vi "Comm_close 1d cdb waveform.vi"(8 "error in (no error)":errorcluster, 11 "WPL Comm (1D CDB) in":refnum<class "WPL Comm (1D CDB).lvclass">) -> (0 "error out":errorcluster)   [LabVIEW 2020, in "Internal Comm Classes.lvlib" / "WPL Comm (1D CDB).lvclass"]
uses:
  WPL Comm (1D CDB).lvclass
  D:/p4/penguin/lvaddon/Veristand/master/src/LabVIEW/vilib/NI VeriStand/Custom Device Waveform API/Internal Comm Classes/WPL Comm/WPL Comm.lvclass
  WPL Comm.lvclass/WPL Comm.ctl
  WPL Comm (1D CDB).lvclass/WPL Comm (1D CDB).ctl
  WPL Command.ctl
  Set ErrorQ on Variant.vi
  Send WPL Command.vi
  WPL Comm.lvclass
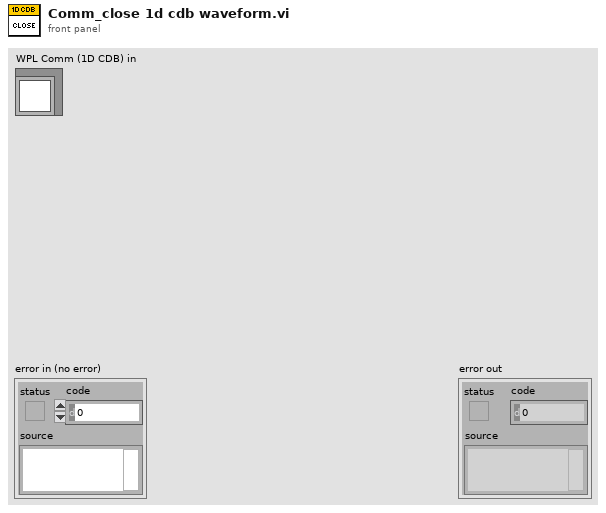
[diagram p1: front panel]
types:
  T1 = typedef "NI_VS Custom Device Waveform API.lvlib/Access mode.ctl" = enum16{"Read", "Write"}
  T2 = typedef "Internal Comm Classes.lvlib/WPL Comm.lvclass/WPL Command.ctl" = enum16{"Register 1D DBL Reader", "Unregister 1D DBL Reader", "Register 1D DBL Writer", "Register 2D DBL Writer", "Unregister 1D DBL Writer", "Unregister 2D DBL Writer", "DBL WFM Start", "WFM 1D DBL Data", "WFM 2D DBL Data", "Shut down", "Handle Error", "Register 1D CDB Reader", "Unregister 1D CDB Reader", "Register 1D CDB Writer", "Unregister 1D CDB Writer", "Register 2D CDB Writer", "Unregister 2D CDB Writer", "WFM 1D CDB Data", "WFM 2D CDB Data", "CDB WFM Start", "Error Shutdown", "Register Streams", "Unregister Streams", "Delete All Streams", "Get WFM DTs", "DBL WFM Multi Start", "CDB WFM Multi Start"}
  T3 = typedef "Internal Comm Classes.lvlib/WPL Comm (1D CDB).lvclass/Waveform 1d cdb read queue.ctl" = refnum<queue>
  T4 = typedef "Internal Comm Classes.lvlib/WPL Comm (1D CDB).lvclass/Waveform 1d cdb queue.ctl" = refnum<queue>
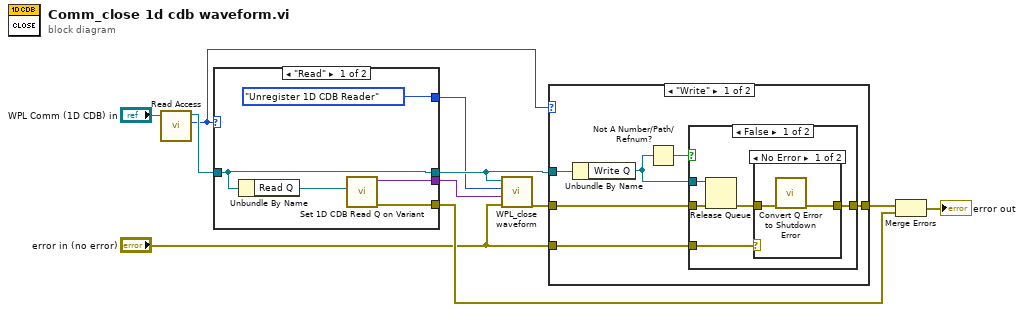
[diagram p0: block diagram]
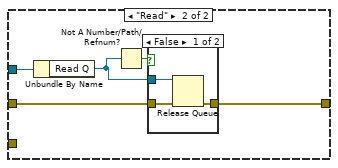
[diagram p4: hidden frame]
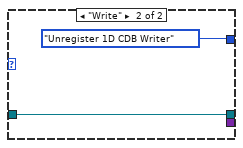
[diagram p6: hidden frame]
diagram:
  n1 = call "Read Access.vi"("WPL Comm in"="WPL Comm (1D CDB) in") -> ("Access"=w6:T1, "WPL Comm out"=w9:refnum<class "WPL Comm (1D CDB).lvclass">)  [unwired: 9 in]
  n2 = case shown="\"Read\"" w6 {
    tunnel: [WPL_Command."Unregister 1D CDB Reader" ("Command") WPL_Command."Unregister 1D CDB Writer" ("Command")] -> w3
    tunnel: w9 -> [w14 w17]
    tunnel: [w14 w17] -> w7
    tunnel: [w15 _] -> w8
    tunnel: [w12 _] -> w2
    frame "Read" {
      n3 = Unbundle By Name(w14) -> ("Read Q"=w13:T3)
      n4 = call "Set 1D CDB Read Q on Variant.vi"("1D CDB Read Q"=w13) -> ("error out"=w15:errorcluster, "Variant out"=w12:variant)  [unwired: 8 in, 1 out]
    }
    frame "Write" {
    }
  }
  n5 = call "WPL_close waveform.vi"("error in (no error)"="error in (no error)", "Variant"=w2, "Command"=w3, "WPL Comm in"=w7) -> ("error out"=w11:errorcluster)  [unwired: 7 in]
  n6 = case shown="\"Write\"" w6 {
    tunnel: w11 -> [w23 w38]
    tunnel: [w20 w37] -> w10
    tunnel: w7 -> [w24 w36]
    tunnel: "error in (no error)" -> [w19 _]
    frame "Write" {
      n7 = Unbundle By Name(w24) -> ("Write Q"=w22:T4)
      n8 = Not A Number/Path/Refnum?(number/path/refnum=w22) -> (NaN/Path/Refnum?=w21:bool)
      n9 = case shown="False" w21 {
        tunnel: w23 -> [w29 w33]
        tunnel: [w26 w33] -> w20
        tunnel: w22 -> [w28 _]
        tunnel: w19 -> [w25 _]
        frame False {
          n10 = Release Queue(queue=w28, error in (no error)=w29) -> (error out=w27:errorcluster)  [unwired: 1 in, 2 out]
          n11 = case shown="No Error" w25 {
            tunnel: w27 -> [w31 w32]
            tunnel: [w30 w32] -> w26
            frame No Error {
              n12 = call "Convert Q Error to Shutdown Error.vi"("error in (no error)"=w31) -> ("error out"=w30:errorcluster)  [unwired: 10 in]
            }
            frame Error {
            }
          }
        }
        frame True {
        }
      }
    }
    frame "Read" {
      n13 = Unbundle By Name(w36) -> ("Read Q"=w35:T3)
      n14 = Not A Number/Path/Refnum?(number/path/refnum=w35) -> (NaN/Path/Refnum?=w34:bool)
      n15 = case shown="False" w34 {
        tunnel: w38 -> [w41 w42]
        tunnel: [w40 w42] -> w37
        tunnel: w35 -> [w39 _]
        frame False {
          n16 = Release Queue(queue=w39, error in (no error)=w41) -> (error out=w40:errorcluster)  [unwired: 1 in, 2 out]
        }
        frame True {
        }
      }
    }
  }
  n17 = Merge Errors(w10, w8) -> (→"error out":errorcluster)
